vi "rs3 Advanced get RAU control3.vi"(8 "error in (no error)":errorcluster, 10 "mode":i32, 11 "device in":u64) -> (0 "error out 2":errorcluster, 1 "error":u64, 2 "ST RAU vector":T1, 3 "Dev out":u64)   [LabVIEW 2017, in "libRealSense3.lvlib"]
doc: "Opens communication to a specific RealSense Device."
uses:
  libRealSense3.lvlib
  realsense2.dll
panel:
  # "RS3 Adv. Get RAU 2"
  # "(C) 2017 Intel Corp.,  AGJ"
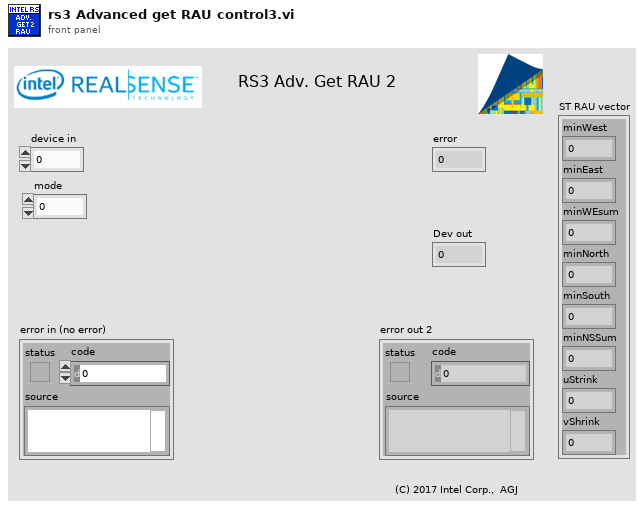
[diagram p1: front panel]
types:
  T1 = cluster{"minWest":u32, "minEast":u32, "minWEsum":u32, "minNorth":u32, "minSouth":u32, "minNSSum":u32, "uStrink":u32, "vShrink":u32}
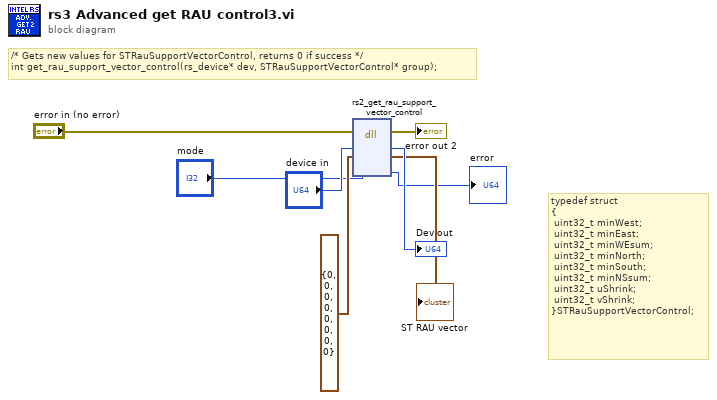
[diagram p0: block diagram]
diagram:
  # "typedef struct\n{\n\tuint32_t minWest;\n\tuint32_t minEast;\n\tuint32_t minWEsum;\n\tuint32_t minNorth;\n\tuint32_t minSouth;\n\tuint32_t minNSsum;\n\tuint32_t uShrink;\n\tuint32_t vShrink;\n}STRauSupportVectorControl;"
  # "/* Gets new values for STRauSupportVectorControl, returns 0 if success */\nint get_rau_support_vector_control(rs_device* dev, STRauSupportVectorControl* group);"
  n1 = dll-call lib="C:/Users/agrunnet/Documents/libRealSense6/realsense2.dll" fn="rs2_get_rau_support_vector_control"(error in="error in (no error)", "device"="device in", "ST RAU vector"=T1 {"minWest"=0, "minEast"=0, "minWEsum"=0, "minNorth"=0, "minSouth"=0, "minNSSum"=0, "uStrink"=0, "vShrink"=0} ("output cluster"), "mode"="mode") -> (error out=→"error out 2":errorcluster, "device"=→"Dev out":u64, "ST RAU vector"=→"ST RAU vector":T1, "error"=→"error":u64)  [unwired: 5 in, 1 out]
